vi "mfd_radio_bat.vi"() -> ()   [LabVIEW 2023]
uses:
  <vilib>/Utility/miscctls.llb/LVBoundsTypeDef.ctl
panel:
  in  "stop":bool
  out "mfd_radio_battery":picture
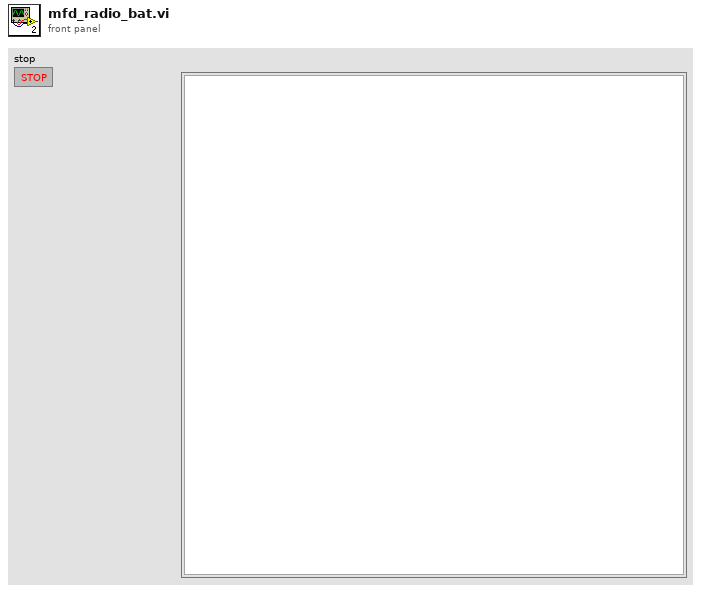
[diagram p1: front panel]
types:
  T1 = cluster{"Font Name:":string, "Size":i16, "Strikeout?":bool, "Italic?":bool, "Underline?":bool, "Outline?":bool, "Shadow?":bool, "Bold?":bool}
  T2 = typedef "LVBoundsTypeDef.ctl" = cluster{"Width":u32, "Height":u32}
  T3 = cluster{"Width":u16, "Style":enum32{"Solid", "Dash", "Dot", "DashDot", "DashDotDot"}}
  T4 = cluster{"left":i16, "top":i16, "right":i16, "bottom":i16}
  T5 = enum16{"User-specified Font", "Application Font", "System Font", "Dialog Font"}
  T6 = cluster{"horizontal":enum16{"left", "center", "right"}, "vertical":enum16{"top", "center", "bottom"}}
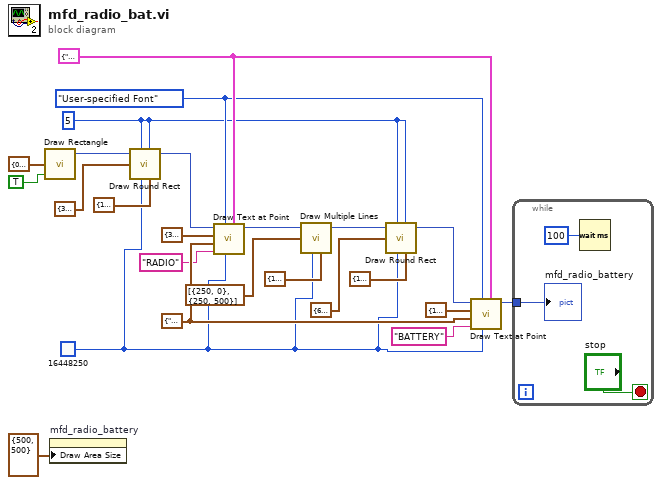
[diagram p0: block diagram]
diagram:
  w18 = T1 {"Font Name:"="r", "Size"=25, "Strikeout?"=FALSE, "Italic?"=FALSE, "Underline?"=FALSE, "Outline?"=FALSE, "Shadow?"=FALSE, "Bold?"=TRUE} ("[user-specified font]")
  w2 = u32 16448250 ("text color(black)")
  w17 = T5."User-specified Font" ("desired font(Application)")
  w19 = T6 {"horizontal"=enum."center", "vertical"=enum."top"} ("alignment(left, top)")
  w1 = i16 5 ("oval height")
  n1 = call <vilib>:"Draw Rectangle.vi"("rect"=T4 {"left"=0, "top"=0, "right"=500, "bottom"=500}, "fill?(F)"=TRUE) -> ("new picture"=w22:picture)  [unwired: 7 in]
  n2 = property on="mfd_radio_battery" class="Pict"("Draw Area Size"=T2 {"Width"=500, "Height"=500}) -> ()  [unwired: 2 in, 2 out]
  n3 = call <vilib>:"Draw Round Rect.vi"("picture"=w22, "oval width"=w1, "rect"=T4 {"left"=334, "top"=19, "right"=413, "bottom"=48}, "color(black)"=w2, "oval height"=w1, "pen"=T3 {"Width"=1, "Style"=enum."Solid"}) -> ("new picture"=w14:picture)  [unwired: 3 in]
  n4 = call <vilib>:"Draw Text at Point.vi"("[user-specified font]"=w18, "text color(black)"=w2, "desired font(Application)"=w17, "text"="RADIO", "alignment(left, top)"=w19, "origin"=cluster{"x":i16, "y":i16} {"x"=375, "y"=22}, "picture"=w14) -> ("new picture"=w13:picture)  [unwired: 3 in, 1 out]
  n5 = call <vilib>:"Draw Multiple Lines.vi"("picture"=w13, "line endpoints"=cluster{"x":i16, "y":i16}[] [{"x"=250, "y"=0}, {"x"=250, "y"=500}], "color(black)"=w2, "pen"=T3 {"Width"=1, "Style"=enum."Solid"} ("pen 2")) -> ("new picture"=w10:picture)  [unwired: 5 in]
  n6 = call <vilib>:"Draw Round Rect.vi"("picture"=w10, "oval width"=w1, "rect"=T4 {"left"=68, "top"=19, "right"=181, "bottom"=48} ("rect 4"), "color(black)"=w2, "oval height"=w1, "pen"=T3 {"Width"=1, "Style"=enum."Solid"}) -> ("new picture"=w5:picture)  [unwired: 3 in]
  n7 = call <vilib>:"Draw Text at Point.vi"("[user-specified font]"=w18, "text color(black)"=w2, "desired font(Application)"=w17, "text"="BATTERY", "alignment(left, top)"=w19, "origin"=cluster{"x":i16, "y":i16} {"x"=125, "y"=22} ("origin 2"), "picture"=w5) -> ("new picture"=w4:picture)  [unwired: 3 in, 1 out]
  n8 = while {
    tunnel: w4 -> [w25]
    stop <- "stop" stop-if-true
    n9 = Wait (ms)(milliseconds to wait=u32 100) -> ()  [unwired: 1 out]
    "mfd_radio_battery" <- w25
  }
